vi "InstrumentCalibration - Load Slope (SubVI).vi"(8 "error in (no error)":errorcluster) -> (0 "error out":errorcluster, 1 "Motor M":dbl[](array[numeric]), 2 "TD MC":dbl[](array[numeric]), 3 "LC MC":dbl[](array[numeric]))   [LabVIEW 2019]
uses:
  Controls/FGV States.ctl
panel:
  out "data":string[][](array[string])
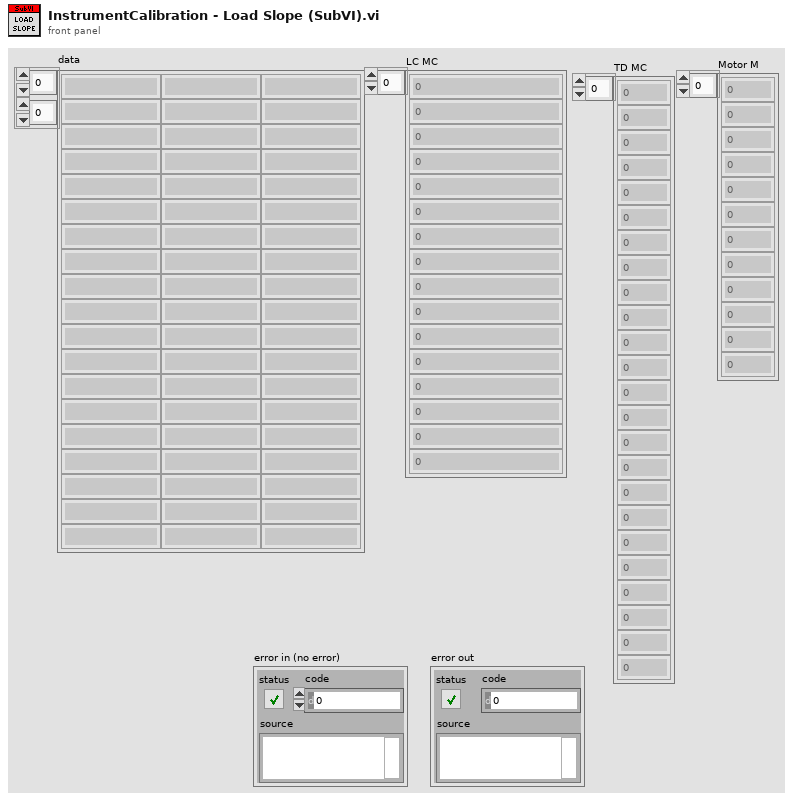
[diagram p1: front panel]
types:
  T1 = typedef "FGV States.ctl" = enum16{"Read", "Write"}
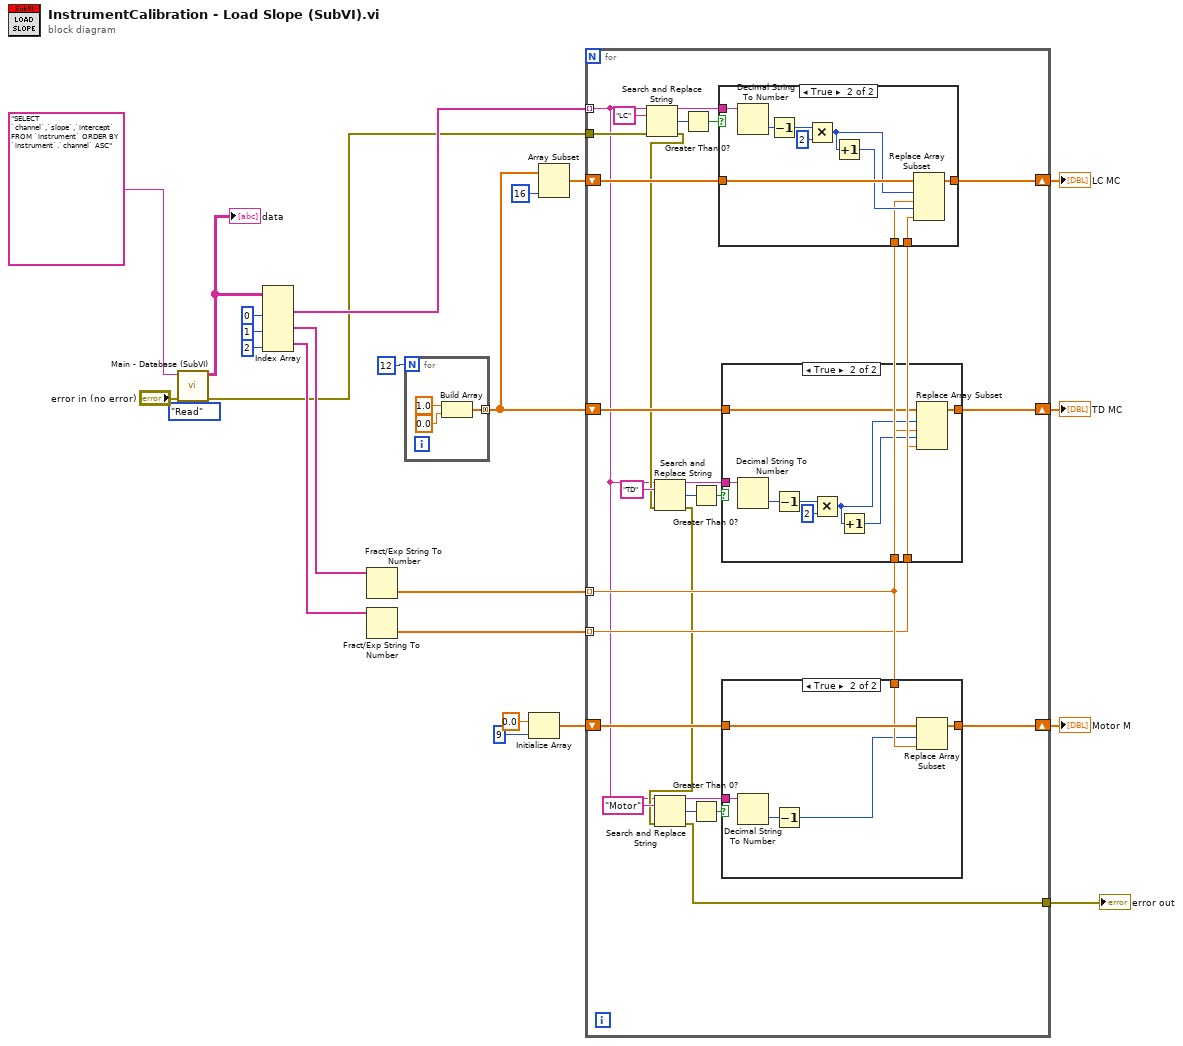
[diagram p0: block diagram]
diagram:
  n1 = call "Main - Database (SubVI).vi"("Enum"=FGV_States."Read", "error in (no error)"="error in (no error)", "SQL query"="SELECT `channel`,`slope`,`intercept` FROM `instrument` ORDER BY `instrument`.`channel` ASC") -> ("error out"=w6:errorcluster, "data"=w22:string[][])  [unwired: 7 in]
  "data" <- w22
  n2 = Index Array(array=w22, index (col) #1=0 ("disabled index (col)"), index (col) #2=1 ("index (col)"), index (col) #3=2 ("index (col)")) -> (element #1=w20:string[], element #2=w13:string[], element #3=w12:string[])  [unwired: 3 in]
  n3 = Fract/Exp String To Number(string=w13) -> (number=w11:dbl[])  [unwired: 3 in, 1 out]
  n4 = Fract/Exp String To Number(string=w12) -> (number=w10:dbl[])  [unwired: 3 in, 1 out]
  n5 = for {
    N: 12 -> [_]
    tunnel: [w25] -> w16 mode=concatenating
    n6 = Build Array(1.0 ("element"), 0.0 ("element")) -> (w25:dbl[])
  }
  n7 = Initialize Array(0.0 ("element"), 9 ("dimension size")) -> (w2:dbl[])
  n8 = Array Subset(array=w16, length=16) -> (w17:dbl[])  [unwired: 1 in]
  n9 = for {
    tunnel: w20 -> [w29] mode=indexing
    shift-right: [w45] -> w9
    shift-left: w17 -> [w46]
    shift-right: [w43] -> w8
    shift-left: w16 -> [w44]
    tunnel: w11 -> [w32] mode=indexing
    tunnel: w10 -> [w31] mode=indexing
    tunnel: w6 -> [w40]
    tunnel: [w28] -> w5
    shift-right: [w33] -> w1
    shift-left: w2 -> [w34]
    n10 = Search and Replace String(input string=w29, search string="LC", error in=w40) -> (result string=w48:string, number of replacements=w50:i32, error out=w39:errorcluster)  [unwired: 5 in, 1 out]
    n11 = Search and Replace String(input string=w29, search string="TD", error in=w39) -> (result string=w47:string, number of replacements=w49:i32, error out=w30:errorcluster)  [unwired: 5 in, 1 out]
    n12 = Search and Replace String(input string=w29, search string="Motor", error in=w30) -> (result string=w37:string, number of replacements=w36:i32, error out=w28:errorcluster)  [unwired: 5 in, 1 out]
    n13 = Greater Than 0?(x=w50) -> (x > 0?=w42:bool)
    n14 = Greater Than 0?(x=w49) -> (x > 0?=w41:bool)
    n15 = Greater Than 0?(x=w36) -> (x > 0?=w38:bool)
    n16 = case shown="True" w42 {
      tunnel: w48 -> [_ w81]
      tunnel: w46 -> [w71 w80]
      tunnel: [w71 w79] -> w45
      tunnel: w32 -> [_ w73]
      tunnel: w31 -> [_ w72]
      frame False {
      }
      frame True {
        n17 = Decimal String To Number(string=w81) -> (number=w76:i32)  [unwired: 2 in, 1 out]
        n18 = Decrement(x=w76) -> (x-1=w78:i32)
        n19 = Multiply(x=w78, y=2) -> (x*y=w75:i32)
        n20 = Increment(x=w75) -> (x+1=w74:i32)
        n21 = Replace Array Subset(array=w80, new element #1=w73, index #1=w75, new element #2=w72, index #2=w74) -> (w79:dbl[])
      }
    }
    n22 = case shown="True" w41 {
      tunnel: w47 -> [_ w70]
      tunnel: w44 -> [w60 w64]
      tunnel: [w60 w63] -> w43
      tunnel: w32 -> [_ w62]
      tunnel: w31 -> [_ w61]
      frame False {
      }
      frame True {
        n23 = Decimal String To Number(string=w70) -> (number=w65:i32)  [unwired: 2 in, 1 out]
        n24 = Decrement(x=w65) -> (x-1=w66:i32)
        n25 = Multiply(x=w66, y=2) -> (x*y=w68:i32)
        n26 = Increment(x=w68) -> (x+1=w69:i32)
        n27 = Replace Array Subset(array=w64, new element #1=w62, index #1=w68, new element #2=w61, index #2=w69) -> (w63:dbl[])
      }
    }
    n28 = case shown="True" w38 {
      tunnel: w37 -> [_ w59]
      tunnel: w34 -> [w53 w57]
      tunnel: [w53 w56] -> w33
      tunnel: w32 -> [_ w55]
      frame False {
      }
      frame True {
        n29 = Decimal String To Number(string=w59) -> (number=w58:i32)  [unwired: 2 in, 1 out]
        n30 = Decrement(x=w58) -> (x-1=w54:i32)
        n31 = Replace Array Subset(array=w57, new element=w55, index=w54) -> (w56:dbl[])
      }
    }
  }
  "LC MC" <- w9
  "TD MC" <- w8
  "error out" <- w5
  "Motor M" <- w1
